vi "Request Addresses Event.vi"(0 "connection info":T1, 1 "DA":refnum<vi>, 2 "Addresses":refnum<vi>, 5 "State Variables":T3, 12 "Error Q":refnum<queue>, 13 "VI Ref":refnum<vi>) -> (4 "connection info":T1, 8 "Address Lookup Table Out":variant)   [LabVIEW 2019, in "J1939 Workspace Shared.lvlib"]
uses:
  J1939 Workspace Shared.lvlib
  Addon/Addon Shared/Types/Error Cluster.ctl
  Addon/Addon Shared/Types/Error Types.ctl
  <vilib>/NI/STM/TCP/TCP Connection Info.ctl
  <vilib>/NI/STM/SubVIs/MetaDataElement.ctl
  Types/Private Data.ctl
  Addon/Addon Shared/J1939 Addon Shared.lvlib
  <vilib>/NI/STM/NI STM.lvlib
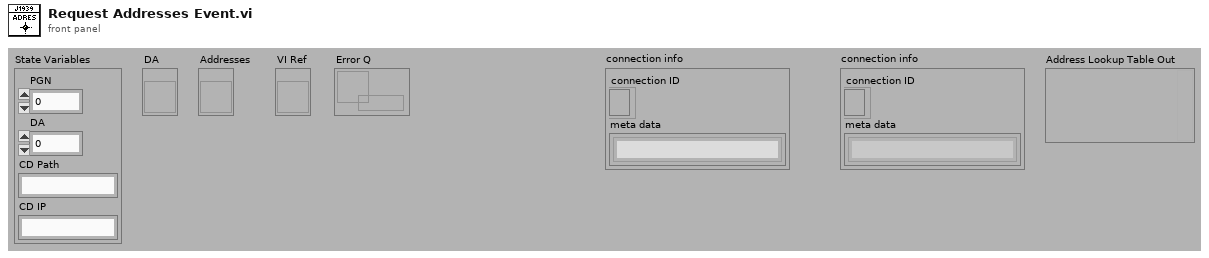
[diagram p1: front panel]
types:
  T1 = typedef "NI STM.lvlib/TCP Connection Info.ctl" = cluster{"connection ID":refnum<k5>, "meta data":T2[]}
  T2 = typedef "NI STM.lvlib/MetaDataElement.ctl" = string
  T3 = typedef "J1939 Workspace Shared.lvlib/Private Data.ctl" = cluster{"PGN":u32, "DA":u8, "CD Path":string, "CD IP":string}
  T4 = typedef "J1939 Addon Shared.lvlib/Error Cluster.ctl" = cluster{"error out":errorcluster, "Enum":T5, "Address":u8, "Timestamp":timestamp}
  T5 = typedef "J1939 Addon Shared.lvlib/Error Types.ctl" = enum16{"Request", "RAW Generation", "Clear Active DTCs", "Clear Previous DTCs", "Addresses", "TLAs", "Get Active DTCs", "Get Previous DTCs", "TCP Connection"}
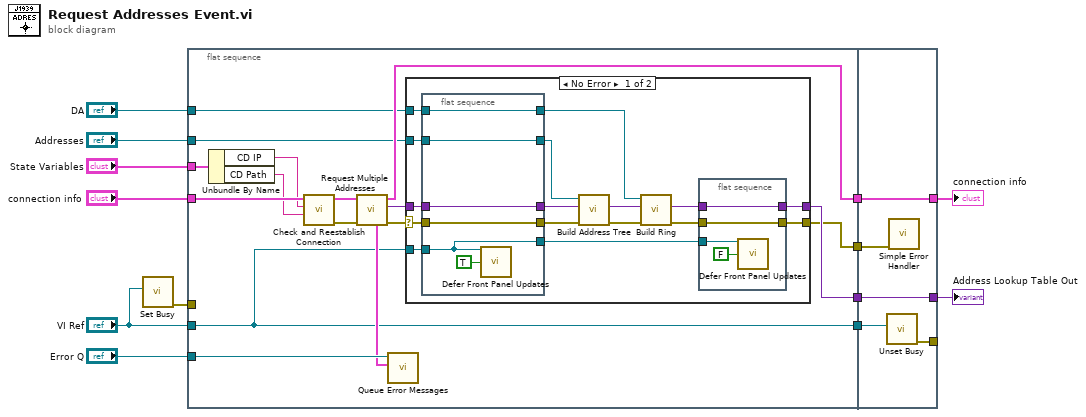
[diagram p0: block diagram]
diagram:
  n1 = call <vilib>:"Set Busy.vi"("VI reference (current VI)"="VI Ref") -> ("error out"=w5:errorcluster)  [unwired: 9 in, 1 out]
  n2 = flat-sequence {
    tunnel: "connection info" -> [w29]
    tunnel: "State Variables" -> [w28]
    tunnel: [w25] -> w13
    tunnel: [w21] -> w12
    tunnel: "Error Q" -> [w20]
    tunnel: [w18] -> w11
    tunnel: w5 -> [_]
    tunnel: "VI Ref" -> [w16]
    tunnel: [w16] -> w3
    tunnel: "Addresses" -> [w15]
    tunnel: "DA" -> [w14]
    tunnel: [w60] -> w9
    tunnel: [w61] -> w8
    tunnel: w13 -> [w61]
    tunnel: w12 -> [w60]
    tunnel: [w59] -> _
    tunnel: w11 -> [w58]
    tunnel: w3 -> [w57]
    frame #0 {
      n3 = Unbundle By Name(w28) -> ("CD IP"=w27:string, "CD Path"=w17:string)
      n4 = call "Check and Reestablish Connection.vi"("CD Path"=w17, "IP Address"=w27, "connection info"=w29) -> ("error out"=w23:errorcluster, "connection info"=w26:T1)  [unwired: 7 in]
      n5 = call "Request Multiple Addresses.vi"("error in (no error)"=w23, "connection info"=w26) -> ("error out"=w24:errorcluster, "variant"=w22:variant, "connection info"=w25:T1, "Error Array"=w19:T4[])  [unwired: 6 in]
      n6 = call "Queue Error Messages.vi"("Error Array"=w19, "queue out"=w20) -> ()  [unwired: 9 in, 1 out]
      n7 = case shown="No Error" w24 {
        selector: w24 -> [w42 w56]
        tunnel: [w37 w56] -> w18
        tunnel: w22 -> [w39 _]
        tunnel: [w34 _] -> w21
        tunnel: w16 -> [w36 _]
        tunnel: w15 -> [w32 _]
        tunnel: w14 -> [w30 _]
        frame No Error {
          n8 = flat-sequence {
            tunnel: [w47] -> w45
            tunnel: w42 -> [w49]
            tunnel: [w50] -> w40
            tunnel: w39 -> [w50]
            tunnel: [w49] -> w38
            tunnel: w36 -> [w48]
            tunnel: [w48] -> w35
            tunnel: w32 -> [w47]
            tunnel: [w46] -> w31
            tunnel: w30 -> [w46]
            frame #0 {
              n9 = call "Defer Front Panel Updates.vi"("This VI"=w48, "Defer Panel Updates"=TRUE) -> ()  [unwired: 13 in, 1 out]
            }
          }
          n10 = call "Build Address Tree.vi"("error in (no error)"=w38, "variant"=w40, "Addresses"=w45) -> ("error out"=w44:errorcluster, "duplicate variant"=w43:variant)  [unwired: 7 in]
          n11 = call "Build Ring.vi"("error in (no error)"=w44, "variant"=w43, "Ring"=w31) -> ("error out"=w41:errorcluster, "duplicate variant"=w33:variant)  [unwired: 7 in]
          n12 = flat-sequence {
            tunnel: w41 -> [w54]
            tunnel: [w54] -> w37
            tunnel: w35 -> [w53]
            tunnel: [w52] -> w34
            tunnel: w33 -> [w52]
            frame #0 {
              n13 = call "Defer Front Panel Updates.vi"("This VI"=w53, "Defer Panel Updates"=FALSE) -> ()  [unwired: 13 in, 1 out]
            }
          }
        }
        frame Error {
        }
      }
    }
    frame #1 {
      n14 = call <vilib>:"Unset Busy.vi"("VI reference (current VI)"=w57) -> ("error out"=w59:errorcluster)  [unwired: 10 in]
      n15 = call <vilib>:"Simple Error Handler.vi"("error in (no error)"=w58) -> ()  [unwired: 4 in, 5 out]
    }
  }
  "Address Lookup Table Out" <- w9
  "connection info" <- w8
